vi "Set_Unit.vi"(0 "VisaCluster":T2, 7 "Unit":T1, 11 "error in (no error)":errorcluster) -> (4 "VisaCluster":T2, 6 "Unit":T1, 8 "Answer":string, 15 "error out":errorcluster)   [LabVIEW 2014, in "FH 55.lvlib"]
doc: "This VI sets the Unit off T, G, A/m.\n\n\nDurch das VI kann die Einheit gewechselt werden (T, G, A/m)."
uses:
  FH 55.lvlib
  TypeDef/VisaCluster.ctl
  TypeDef/Unit.ctl
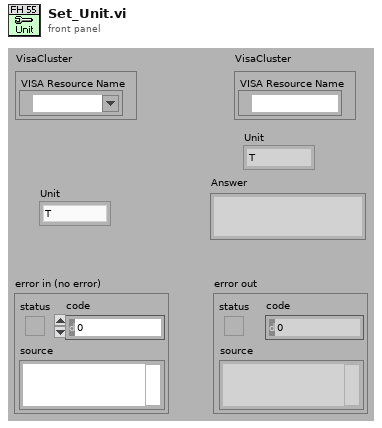
[diagram p1: front panel]
types:
  T1 = typedef "FH 55.lvlib/Unit.ctl" = enum16{"T", "G", "A/m"}
  T2 = typedef "FH 55.lvlib/VisaCluster.ctl" = cluster{"VISA Resource Name":refnum<visa-resource-name>}
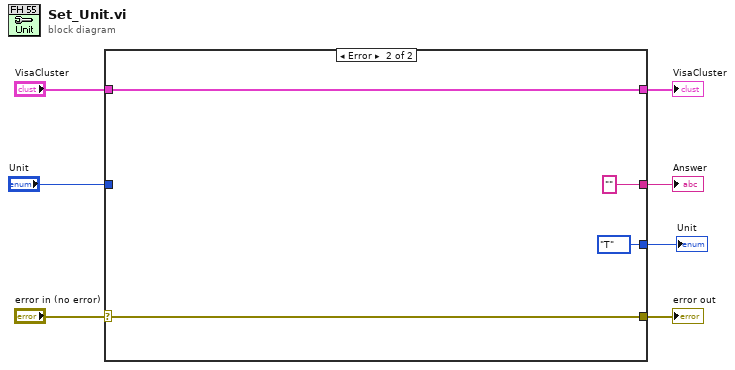
[diagram p0: block diagram]
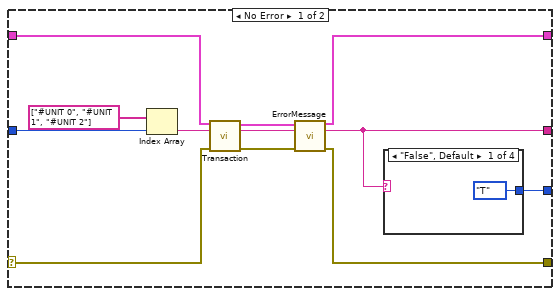
[diagram p2: hidden frame]
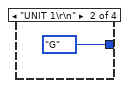
[diagram p3: hidden frame]
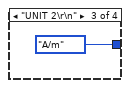
[diagram p4: hidden frame]
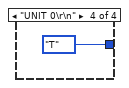
[diagram p5: hidden frame]
diagram:
  n1 = case shown="Error" "error in (no error)" {
    selector: "error in (no error)" -> [w16 w26]
    tunnel: "VisaCluster" -> [w17 w27]
    tunnel: "Unit" -> [w12 _]
    tunnel: [w19 w27] -> w3
    tunnel: [w18 w26] -> w5
    tunnel: [w9 ""] -> w4
    tunnel: [w8 Unit."T" ("Unit 3")] -> w1
    frame No Error {
      n2 = Index Array(array=string[] ["#UNIT 0", "#UNIT 1", "#UNIT 2"], index=w12) -> (element=w10:string)
      n3 = call "Transaction.vi"("VisaCluster"=w17, "Command"=w10, "error in (no error)"=w16) -> ("VisaCluster"=w13:T2, "Answer"=w14:string, "error out"=w15:errorcluster)  [unwired: 9 in, 1 out]
      n4 = call "ErrorMessage.vi"("VisaCluster"=w13, "Message In"=w14, "error in (no error)"=w15) -> ("VisaCluster"=w19:T2, "Message Out"=w9:string, "error out"=w18:errorcluster)  [unwired: 10 in]
      n5 = case shown="\"False\", Default" w9 {
        tunnel: [Unit."T" ("Unit 3") Unit."G" ("Unit 3") Unit."A/m" ("Unit 3") Unit."T" ("Unit 3")] -> w8
        frame "False", Default {
        }
        frame "UNIT 1\r\n" {
        }
        frame "UNIT 2\r\n" {
        }
        frame "UNIT 0\r\n" {
        }
      }
    }
    frame Error {
    }
  }
  "error out" <- w5
  "Answer" <- w4
  "VisaCluster" <- w3
  "Unit" <- w1
